vi "Create Event Control.vi"(8 "Error In":errorcluster, 11 "Node Refnum in":refnum<vi>) -> (0 "Error Out":errorcluster, 2 "Control":refnum<vi>, 3 "Node Refnum out":refnum<vi>)   [LabVIEW 2011, in "Generator.lvlib"]
doc: "This VI creates a control of the event type and returns the reference to it."
uses:
  Generator.lvlib
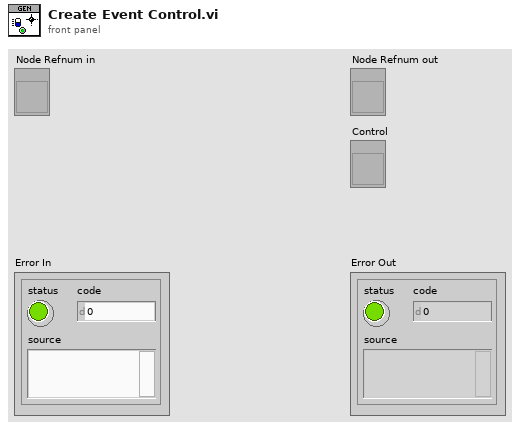
[diagram p1: front panel]
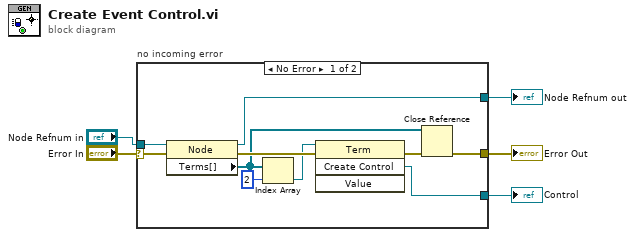
[diagram p0: block diagram]
diagram:
  n1 = case "no incoming error" shown="No Error" "Error In" {
    selector: "Error In" -> [w10 w17]
    tunnel: [w8 w17] -> w4
    tunnel: "Node Refnum in" -> [w9 w16]
    tunnel: [w7 w16] -> w2
    tunnel: [w6 _] -> w1
    frame No Error {
      n2 = property class="Node"(reference=w9, error in=w10) -> (reference out=w7:refnum<vi>, error out=w14:errorcluster, "Terms[]"=w11:refnum<vi>[])
      n3 = Index Array(array=w11, index=2) -> (element=w13:refnum<vi>)
      n4 = invoke class="Term" method="Create Control"(reference=w13, error in=w14) -> (error out=w12:errorcluster, "Create Control"=w6:refnum<vi>)  [unwired: 2 in, 2 out]
      n5 = Close Reference(reference=w11, error in (no error)=w12) -> (error out=w8:errorcluster)
    }
    frame Error {
    }
  }
  "Error Out" <- w4
  "Node Refnum out" <- w2
  "Control" <- w1
